vi "EEISysLink Test Harness.vi"() -> ()   [LabVIEW 2016]
uses:
  Controls/SL Tag Value.ctl
  Controls/SL Tag Data Type.ctl
  EEISysLink.lvclass
  Controls/SL Tag Scope.ctl
  Controls/SL Tag Type.ctl
panel:
  out "Tag Values 2":T1[](array[typedef])
  out "Tag Server Updates":i32
  in  "error in (no error)":errorcluster
  out "Tag Values":T1[](array[typedef])
  out "Tag Error Count":i32
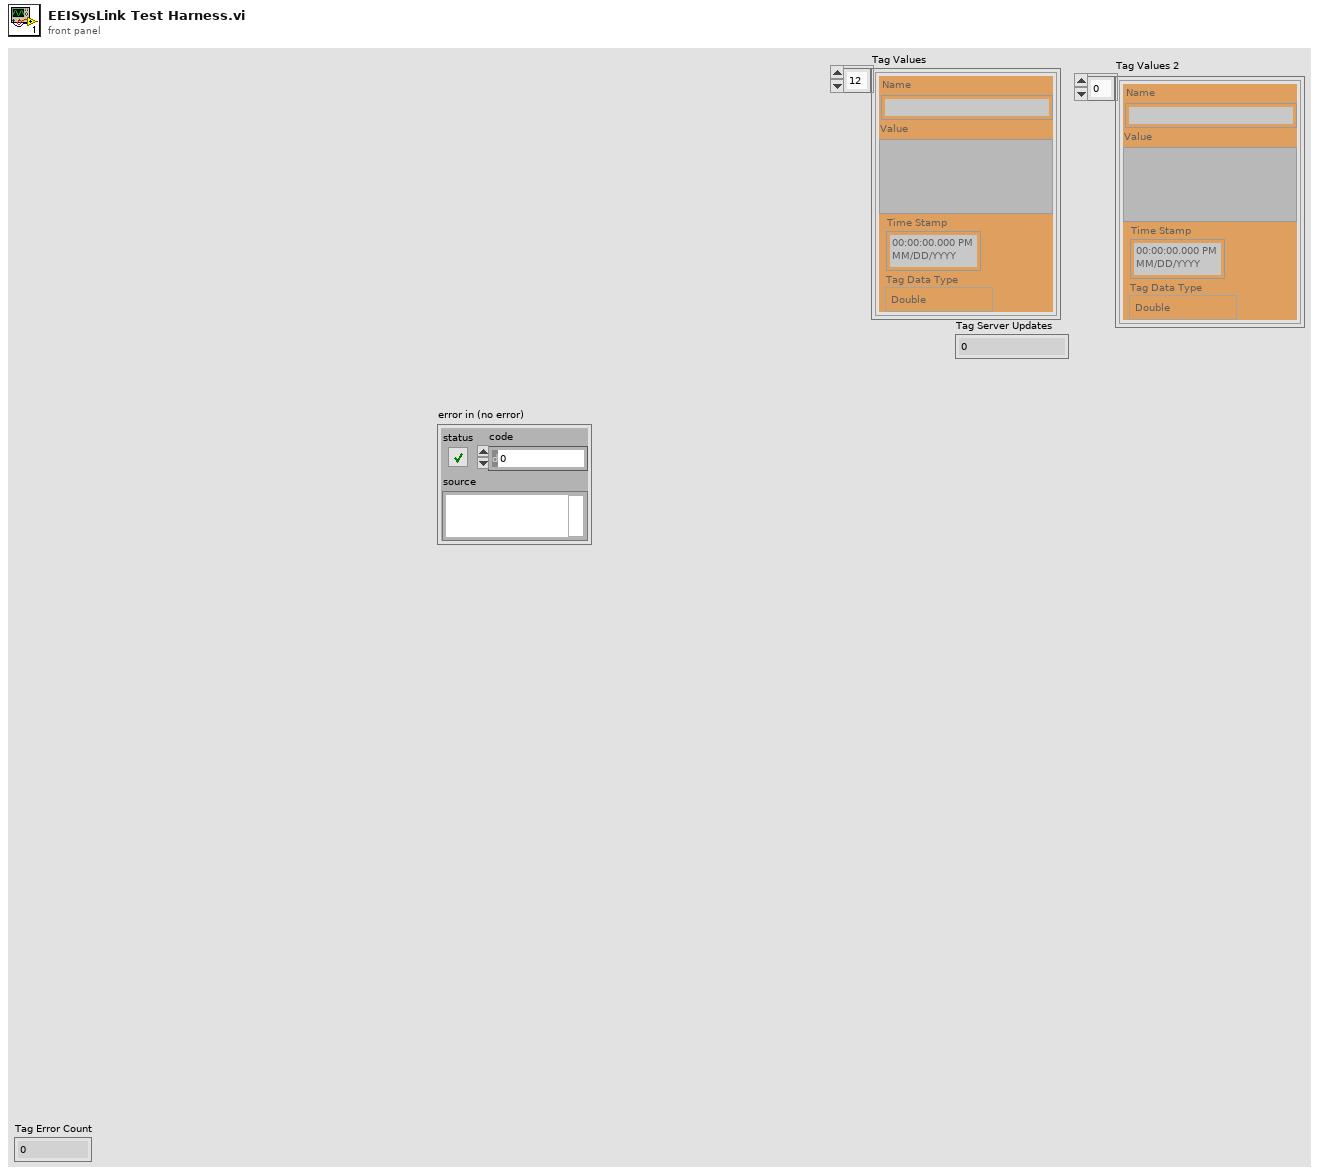
[diagram p1: front panel]
types:
  T1 = typedef "SL Tag Value.ctl" = cluster{"Value":variant, "Time Stamp":timestamp, "Tag Data Type":T2, "Name":string}
  T2 = typedef "EEISysLink.lvclass/SL Tag Data Type.ctl" = enum16{"Double", "Integer", "String", "Boolean", "Waveform"}
  T3 = typedef "EEISysLink.lvclass/SL Tag Type.ctl" = enum16{"All", "Supervisor", "Worker"}
  T4 = typedef "EEISysLink.lvclass/SL Tag Scope.ctl" = enum16{"Local", "Server"}
  T5 = typedef "EEISysLink.lvclass/SL Tag Properties.ctl" = cluster{"Data Type":T2, "Name":string, "Description":string, "Interpolation Method":T6, "Unit of Measure":T7, "Maximum Interpolation":string, "Type":T3}
  T6 = typedef "EEISysLink.lvclass/SL Tag Interpolation Method.ctl" = enum16{"linear", "pilinear", "step"}
  T7 = typedef "EEISysLink.lvclass/SL Tag Unit of Measure.ctl" = enum16{"no units", "Second", "Hour", "Minute", "Day", "Year", "Month", "Week", "Foot", "Yard", "Meter", "Centimeter", "Inch", "Mile", "Nautical Mile", "Miles per Hour", "Meters per second", "Square meter", "Cubic meter", "Cubic centimeter", "Cubic inch", "Liter", "Gallon", "Gallons dry US", "Gallon UK", "Percent", "Revolutions per minute", "Revolution", "Degree angle", "Astronomical Unit", "Atom", "Atomic mass", "Bar", "Byte", "C (speed of light)", "Curie", "Decibel", "Electron Volt", "Ounce", "Knot", "G", "Grade", "Are", "Hectare", "Faraday", "Franklin", "Gilbert", "Erg", "Lambert", "Maxwell", "Gauss", "Electron mass", "Kilogram force", "Pound force", "Rad", "Centiradian", "Sphere", "Mach", "Fluid Ounces", "Fluid Ounces UK", "Fahrenheit", "Celsius", "Kelvin", "Rankine", "Gram", "Kilogram", "Pound", "Short/US Ton", "Long/UK ton", "Metric ton", "Mole", "Pounds per square inch", "Inches water column", "Torr", "Millitorr", "Millimeter mercury", "Inches mercury", "Bar (2)", "Atmosphere", "Pascal", "Watt", "kiloWatt", "Horsepower", "Kilowatt Hour", "British thermal units", "Millions of BTU", "Ampere", "Candela", "Radian", "Steradian", "Bit", "Hertz", "Newton", "Joule", "Coulomb", "Volt", "Farad", "Ohm", "Siemens", "Weber", "Tesla", "Henry", "Lumen", "Lux", "Becqueral", "Gray", "Sievert", "Katal", "Angstrom", "Light Year", "Parsec", "Point", "Pixel", "Dyne", "Kilogram force (2)", "Pound force (2)", "Rem", "Rutherford", "Roentgen"}
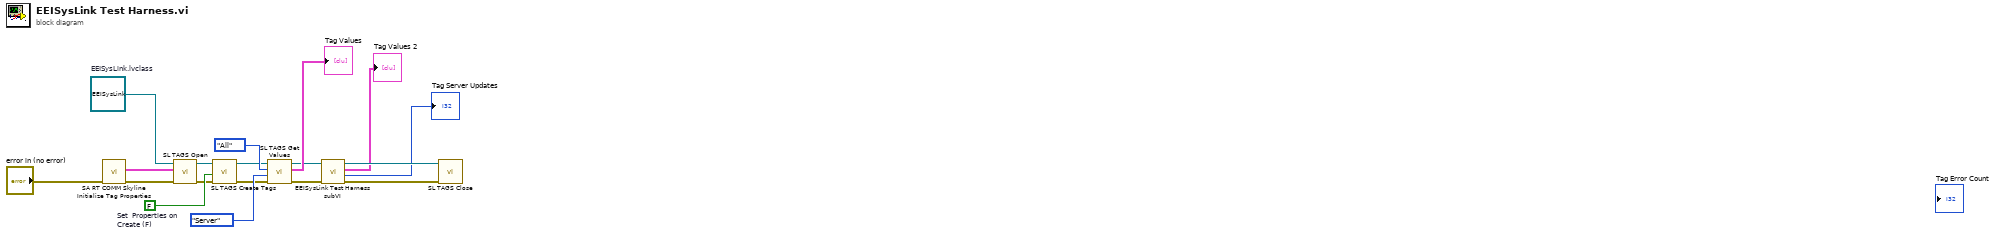
[diagram p0: block diagram]
diagram:
  w9 = refnum<class "EEISysLink.lvclass"> refnum  # EEISysLink.lvclass
  w12 = FALSE  # Set  Properties on Create (F)
  n1 = call "SA RT COMM Skyline Initialize Tag Properties.vi"("error in (no error)"="error in (no error)") -> ("error out"=w8:errorcluster, "Tag Properties"=w18:T5[])  [unwired: 9 in]
  n2 = call-dynamic "SL TAGS Open.vi"("error in (no error)"=w8, "Tag Properties"=w18, "EEISysLink in"=w9) -> ("error out"=w10:errorcluster, "EEISysLink out"=w11:refnum<class "EEISysLink.lvclass">)  [unwired: 7 in]
  n3 = call-dynamic "SL TAGS Create Tags.vi"("error in (no error)"=w10, "Set  Properties on Create (F)"=w12, "EEISysLink in"=w11) -> ("error out"=w14:errorcluster, "EEISysLink out"=w13:refnum<class "EEISysLink.lvclass">)  [unwired: 7 in]
  n4 = call-dynamic "SL TAGS Get Values.vi"("error in (no error)"=w14, "Tag Scope"=SL_Tag_Scope."Server", "Tag Type"=SL_Tag_Type."All", "EEISysLink in"=w13) -> ("error out"=w3:errorcluster, "Tag Values"=→"Tag Values":T1[], "EEISysLink out"=w2:refnum<class "EEISysLink.lvclass">)  [unwired: 5 in]
  n5 = call "EEISysLink Test Harness subVI.vi"("error in (no error)"=w3, "EEISysLink in"=w2) -> ("error out"=w5:errorcluster, "Tag Server Updates"=→"Tag Server Updates":i32, "Tag Values 2"=→"Tag Values 2":T1[], "EEISysLink out"=w6:refnum<class "EEISysLink.lvclass">)  [unwired: 6 in]
  n6 = call-dynamic "SL TAGS Close.vi"("error in (no error)"=w5, "EEISysLink in"=w6) -> ()  [unwired: 8 in, 2 out]
